vi "Sr830 CheckStatus.vi"(6 "error in (no error)":errorcluster, 7 "Ask Correction":bool, 8 "Autoscale":bool, 9 "Ressource VISA In":refnum<visa-resource-name>="GPIB0::8::INSTR") -> (0 "error out":errorcluster, 1 "Warning":bool, 2 "Ask Correction Out":bool, 3 "Ressource VISA Out":refnum<visa-resource-name>="GPIB0::8::INSTR", 4 "Reprise":bool, 5 "Status Byte":bool[](array[boolean]))   [LabVIEW 2010]
panel:
  # "Input/Amplifier OVL"
  # "Time Constant Filter OVL"
  # "Output OVL"
  # "Pll unlck"
  # "Time constant Changed"
  # "Trigger"
  # "unused"
  # "Freq Range Changed"
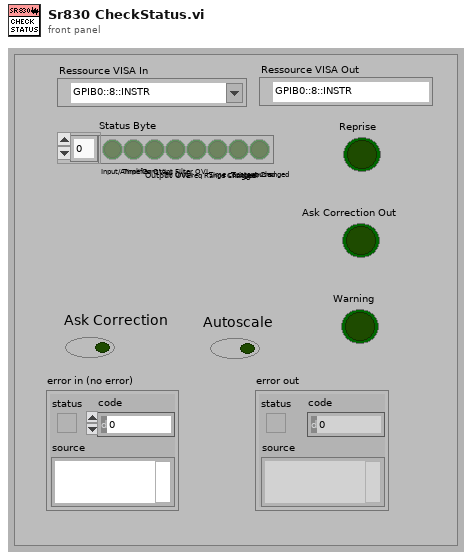
[diagram p1: front panel]
types:
  T1 = enum16{"Read Status", "Status Message", "Find Error", "PLL", "Overload", "Change Scale"}
  T2 = enum32{"Invalid", "Standard", "Closed", "Hidden", "Minimized", "Maximized"}
  T3 = enum16{"Left Button", "Center Button", "Right Button", "Window Close"}
  T4 = enum32{"Bad", "Idle", "Run top level", "Running"}
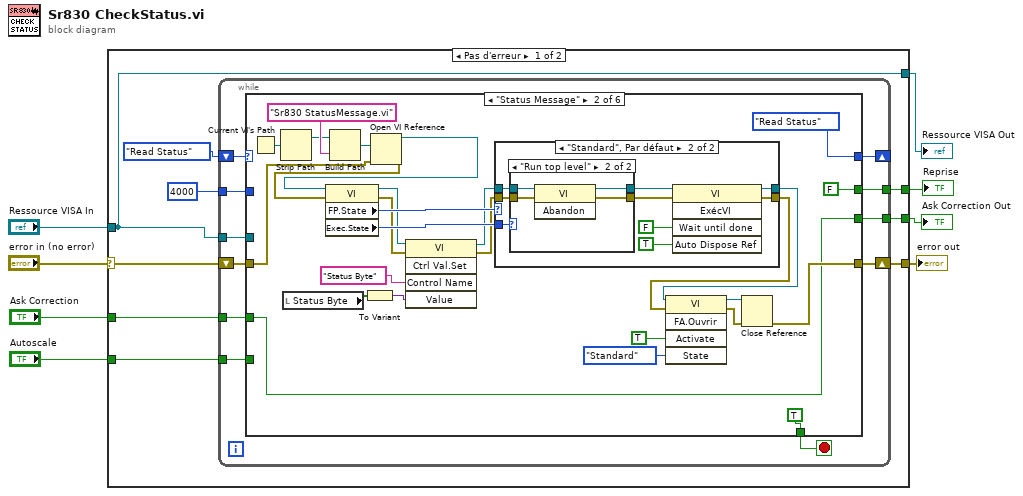
[diagram p0: block diagram]
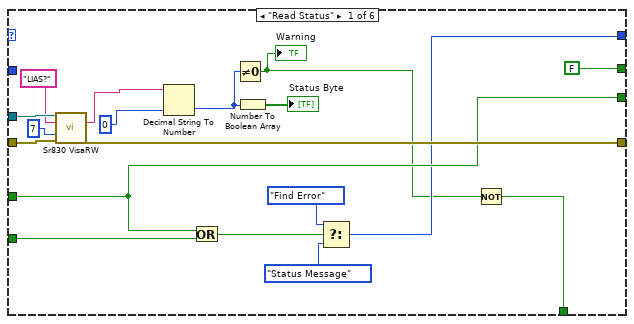
[diagram p2: hidden frame]
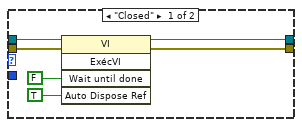
[diagram p3: hidden frame]
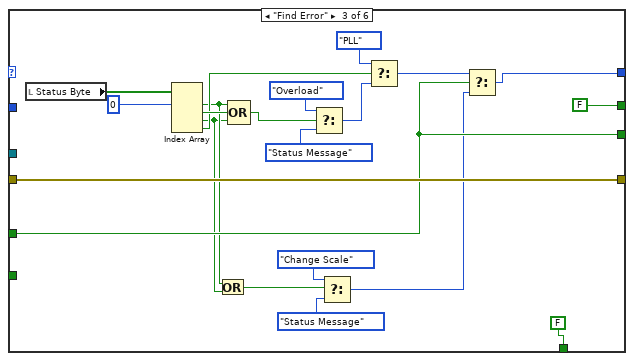
[diagram p5: hidden frame]
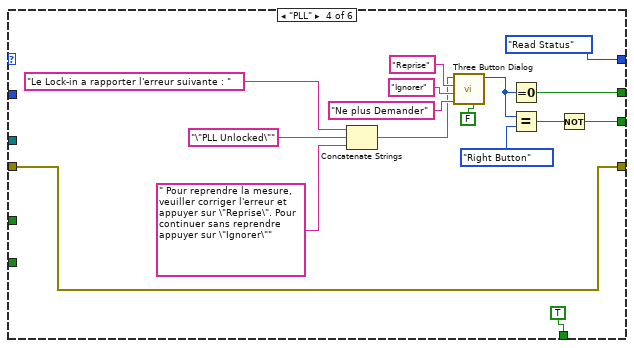
[diagram p6: hidden frame]
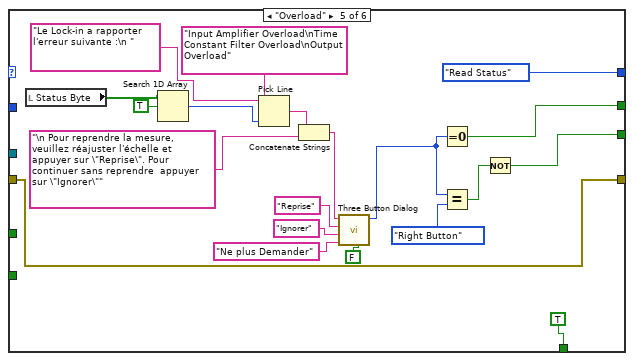
[diagram p7: hidden frame]
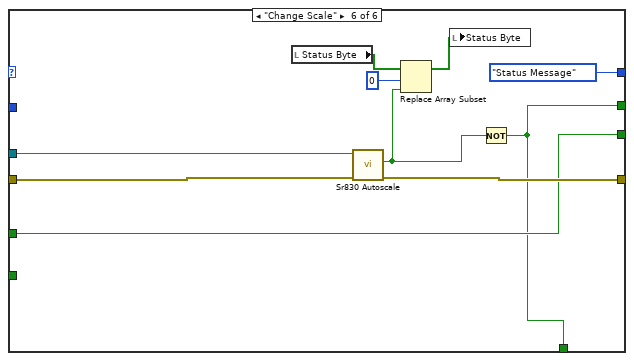
[diagram p8: hidden frame]
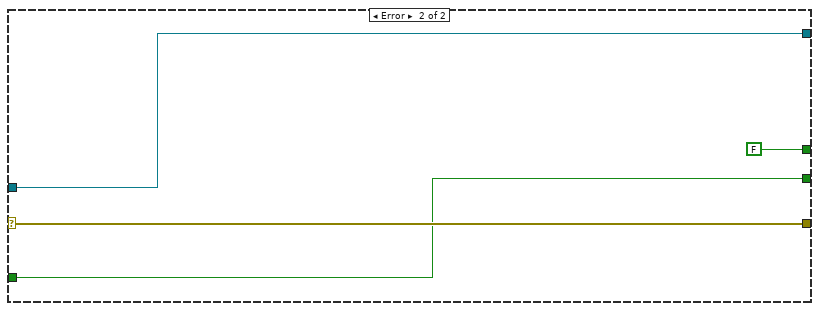
[diagram p9: hidden frame]
diagram:
  n1 = case shown="Pas d'erreur" "error in (no error)" {
    selector: "error in (no error)" -> [w13 w165]
    tunnel: [w16 w165] -> w7
    tunnel: "Autoscale" -> [w15 _]
    tunnel: "Ask Correction" -> [w14 w163]
    tunnel: [w11 FALSE] -> w3
    tunnel: [w10 w163] -> w4
    tunnel: "Ressource VISA In" -> [w9 w162]
    tunnel: [w9 w162] -> w1
    frame No Error {
      n2 = while {
        shift-right: [w23] -> _
        shift-left: T1."Read Status" -> [w28]
        shift-right: [w26] -> w16
        shift-left: w13 -> [w27]
        tunnel: 4000 ("timeout ms (488.2 global)") -> [w25]
        tunnel: w15 -> [w22]
        tunnel: w14 -> [w21]
        tunnel: w9 -> [w20]
        tunnel: [w19] -> w11
        tunnel: [w18] -> w10
        stop <- w24 stop-if-true
        n3 = case shown="\"Status Message\"" w28 {
          tunnel: w27 -> [w46 w60 w109 w120 w150 w161]
          tunnel: [w45 w61 w109 w120 w150 w160] -> w26
          tunnel: w25 -> [_ _ _ _ _ _]
          tunnel: [w32 TRUE FALSE TRUE TRUE w157] -> w24
          tunnel: [w34 T1."Read Status" w102 T1."Read Status" T1."Read Status" T1."Status Message"] -> w23
          tunnel: w22 -> [w36 _ _ _ _ _]
          tunnel: w21 -> [w37 w55 w106 _ _ w159]
          tunnel: w20 -> [w44 _ _ _ _ w152]
          tunnel: [w37 w55 w106 w117 w148 w159] -> w18
          tunnel: [FALSE FALSE FALSE w119 w149 w157] -> w19
          frame "Read Status" {
            n4 = call <userlib>:"Sr830 VisaRW.vi"("VISA Rsrc"=w44, "ChaineCom"="LIAS?", "Nbcaract"=u32 7, "error in (no error)"=w46) -> ("ChaineRep"=w31:string, "error out"=w45:errorcluster)  [unwired: 8 in, 2 out]
            n5 = Decimal String To Number(string=w31, default (0L)=u8 0 ("default (0 I32)")) -> (number=w30:u8)  [unwired: 1 in, 1 out]
            n6 = Or(x=w37, y=w36) -> (x .or. y?=w35:bool)
            n7 = Not Equal To 0?(x=w30) -> (x != 0?=w33:bool)
            "Warning" <- w33
            n8 = Number To Boolean Array(number=w30) -> (Boolean array=→"Status Byte":bool[])
            n9 = Select(t=T1."Find Error", s=w35, f=T1."Status Message") -> (s? t:f=w34:T1)
            n10 = Not(x=w33) -> (.not. x?=w32:bool)
          }
          frame "Status Message" {
            n11 = Current VI's Path() -> (path=w71:path)
            n12 = Strip Path(path=w71) -> (stripped path=w72:path)  [unwired: 1 out]
            n13 = local read "Status Byte"() -> (w58:bool[])
            n14 = Build Path(base path=w72, name or relative path="Sr830 StatusMessage.vi" ("nom ou chemin relatif")) -> (appended path=w67:path)
            n15 = To Variant(anything=w58) -> (Variant=w64:variant)
            n16 = Open VI Reference(vi path=w67, error in (no error)=w60) -> (vi reference=w68:refnum<vi>, error out=w59:errorcluster)  [unwired: 4 in]
            n17 = property class="VI"(reference=w68, error in=w59) -> (reference out=w48:refnum<vi>, error out=w49:errorcluster, "FP.State"=w69:T2, "Exec.State"=w70:T4)
            n18 = invoke class="VI" method="Ctrl Val.Set"(reference=w48, error in=w49, "Control Name"="Status Byte" ("Nom de la commande"), "Value"=w64) -> (reference out=w50:refnum<vi>, error out=w51:errorcluster)  [unwired: 1 in, 3 out]
            n19 = case shown="\"Standard\", Par défaut" w69 {
              tunnel: [w76 w85] -> w52
              tunnel: w50 -> [w77 w83]
              tunnel: w70 -> [_ w84]
              tunnel: w51 -> [w75 w82]
              tunnel: [w74 w80] -> w53
              frame "Closed" {
                n20 = invoke class="VI" method="ExécVI"(reference=w77, error in=w75, "Wait until done"=FALSE ("Attendre la fin"), "Auto Dispose Ref"=TRUE ("Supprimer la référence automatiquement")) -> (reference out=w76:refnum<vi>, error out=w74:errorcluster)  [unwired: 1 in, 3 out]
              }
              frame "Standard", Default {
                n21 = case shown="\"Run top level\"" w84 {
                  tunnel: [w90 w94] -> w86
                  tunnel: w83 -> [w90 w93]
                  tunnel: w82 -> [w89 w92]
                  tunnel: [w89 w91] -> w81
                  frame "Idle", Default {
                  }
                  frame "Run top level" {
                    n22 = invoke class="VI" method="Abandon"(reference=w93, error in=w92) -> (reference out=w94:refnum<vi>, error out=w91:errorcluster)  [unwired: 1 in, 1 out]
                  }
                }
                n23 = invoke class="VI" method="ExécVI"(reference=w86, error in=w81, "Wait until done"=FALSE ("Attendre la fin"), "Auto Dispose Ref"=TRUE ("Supprimer la référence automatiquement")) -> (reference out=w85:refnum<vi>, error out=w80:errorcluster)  [unwired: 1 in, 3 out]
              }
            }
            n24 = invoke class="VI" method="FA.Ouvrir"(reference=w52, error in=w53, "Activate"=TRUE ("Activer ?"), "State"=T2."Standard" ("État")) -> (reference out=w63:refnum<vi>, error out=w62:errorcluster)  [unwired: 1 in, 3 out]
            n25 = Close Reference(reference=w63, error in (no error)=w62) -> (error out=w61:errorcluster)
          }
          frame "Find Error" {
            n26 = local read "Status Byte"() -> (w114:bool[])
            n27 = Index Array(array=w114, index #1=0 ("indice")) -> (element #1=w97:bool, element #2=w113:bool, element #3=w96:bool, element #4=w99:bool)  [unwired: 3 in]
            n28 = Or(x=w97, y=w96) -> (x .or. y?=w95:bool)
            n29 = Compound Arithmetic op=OR(w97, w113, w96) -> (w98:bool)
            n30 = Select(t=T1."Overload", s=w98, f=T1."Status Message") -> (s? t:f=w112:T1)
            n31 = Select(t=T1."Change Scale", s=w95, f=T1."Status Message") -> (s? t:f=w103:T1)
            n32 = Select(t=T1."PLL", s=w99, f=w112) -> (s? t:f=w105:T1)
            n33 = Select(t=w105, s=w106, f=w103) -> (s? t:f=w102:T1)
          }
          frame "PLL" {
            n34 = Concatenate Strings("Le Lock-in a rapporter l'erreur suivante : ", "\"PLL Unlocked\"", " Pour reprendre la mesure, veuiller corriger l'erreur et appuyer sur \"Reprise\". Pour continuer sans reprendre  appuyer sur \"Ignorer\"" ("message")) -> (w125:string)
            n35 = call <vilib>:"Three Button Dialog.vi"("Allow user to close window? (TRUE)"=FALSE, "Right Button Text (\"Cancel\")"="Ne plus Demander" ("F button name (\"Cancel\")"), "Center Button Text (\"No\")"="Ignorer" ("F button name (\"Cancel\")"), "Left Button Text (\"Yes\")"="Reprise" ("T button name (\"OK\")"), "message"=w125) -> ("Which Button?"=w123:T3)  [unwired: 6 in]
            n36 = Equal To 0?(x=w123) -> (x = 0?=w119:bool)
            n37 = Equal?(x=w123, y=T3."Right Button") -> (x = y?=w118:bool)
            n38 = Not(x=w118) -> (.not. x?=w117:bool)
          }
          frame "Overload" {
            n39 = local read "Status Byte"() -> (w139:bool[])
            n40 = Search 1D Array(1D array=w139, element=TRUE ("élément")) -> (index of element=w135:i32)  [unwired: 1 in]
            n41 = Pick Line(string ("")="Le Lock-in a rapporter l'erreur suivante :\n " ("message"), multi-line string="Input Amplifier Overload\nTime Constant Filter Overload\nOutput Overload" ("message"), line index=w135) -> (output string=w134:string)
            n42 = Concatenate Strings(w134, "\n Pour reprendre la mesure, veuillez réajuster l'échelle et appuyer sur \"Reprise\". Pour continuer sans reprendre  appuyer sur \"Ignorer\"" ("message")) -> (w132:string)
            n43 = call <vilib>:"Three Button Dialog.vi"("Allow user to close window? (TRUE)"=FALSE, "Right Button Text (\"Cancel\")"="Ne plus Demander" ("F button name (\"Cancel\")"), "Center Button Text (\"No\")"="Ignorer" ("F button name (\"Cancel\")"), "Left Button Text (\"Yes\")"="Reprise" ("T button name (\"OK\")"), "message"=w132) -> ("Which Button?"=w141:T3)  [unwired: 6 in]
            n44 = Equal To 0?(x=w141) -> (x = 0?=w149:bool)
            n45 = Equal?(x=w141, y=T3."Right Button") -> (x = y?=w140:bool)
            n46 = Not(x=w140) -> (.not. x?=w148:bool)
          }
          frame "Change Scale" {
            n47 = local read "Status Byte"() -> (w156:bool[])
            n48 = call <userlib>:"Sr830 Autoscale.vi"("error in"=w161, "Ressource VISA"=w152) -> ("error out"=w160:errorcluster, "OverRanged"=w154:bool)  [unwired: 2 in, 2 out]
            n49 = Replace Array Subset(array=w156, new element=w154, index=0 ("indice")) -> (w153:bool[])
            n50 = local write "Status Byte"(w153) -> ()
            n51 = Not(x=w154) -> (.not. x?=w157:bool)
          }
        }
      }
    }
    frame Error {
    }
  }
  "error out" <- w7
  "Reprise" <- w3
  "Ask Correction Out" <- w4
  "Ressource VISA Out" <- w1
